vi "Write Version String.vi"(8 "error in (no error)":errorcluster, 10 "Version String":string, 11 "Change Log in":refnum<class "Change Log.lvclass">) -> (0 "error out":errorcluster, 3 "Change Log out":refnum<class "Change Log.lvclass">)   [LabVIEW 2015, in "Change Log.lvlib" / "Change Log.lvclass"]
uses:
  Change Log.lvclass
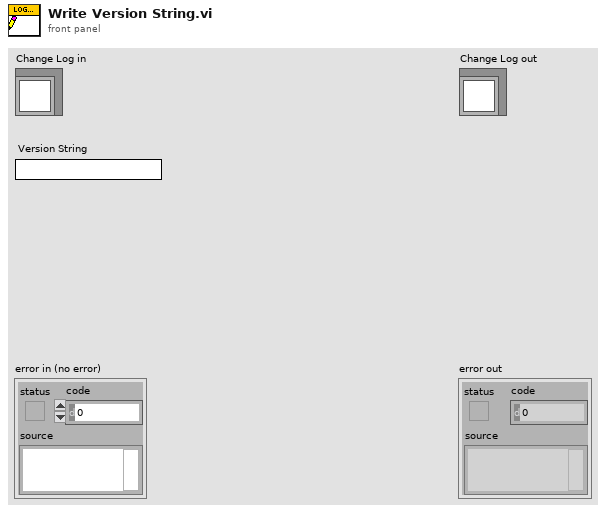
[diagram p1: front panel]
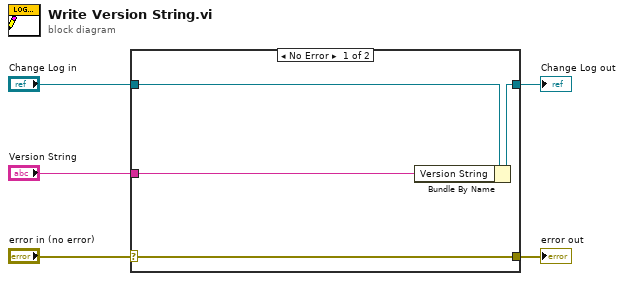
[diagram p0: block diagram]
diagram:
  n1 = case shown="No Error" "error in (no error)" {
    selector: "error in (no error)" -> [w9 w10]
    tunnel: [w9 w10] -> w4
    tunnel: [w7 w11] -> w2
    tunnel: "Change Log in" -> [w8 w11]
    tunnel: "Version String" -> [w6 _]
    frame No Error {
      n2 = Bundle By Name(cluster=w8, "Version String"=w6) -> (w7:refnum<class "Change Log.lvclass">)
    }
    frame Error {
    }
  }
  "error out" <- w4
  "Change Log out" <- w2
